vi "GlobalGUI.vi"() -> ()   [LabVIEW 2014]
panel:
  in  "PortNumber":string="51717"
  in  "IPAddresse":string="192.168.1.22"
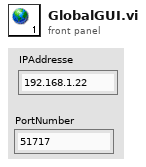
[diagram p1: front panel]
diagram:
